vi "Process.vi"(0 "reference in":refnum<class "ACIR_EIS.lvclass">, 5 "error in":errorcluster) -> (14 "reference out":refnum<class "ACIR_EIS.lvclass">, 19 "error out":errorcluster)   [LabVIEW 2023, in "ACIR_EIS.lvclass"]
uses:
  ACIR_EIS.lvclass
  ACIR_EIS.lvclass/ACIR_EIS.ctl
  <vilib>/Utility/SystemLogging/NI_SystemLogging.lvlib
  EIS Mode.ctl
  EIS Parameters.ctl
  Logger_class/Logger.lvclass
  <userlib>/_OpenG.lib/time/time.llb/openg_time.lvlib
  <vilib>/Utility/NIReport.llb/NI_report.lvclass
  <vilib>/Utility/NIReport.llb/Report Type.ctl
  <vilib>/Utility/NIReport.llb/NI_ReportGenerationCore.lvlib
  builds/PowerModuleInterface/PowerModuleInterface.lvlibp/Classes/PowerModule_interface/PowerModuleInterface.lvclass
  <vilib>/printing/OpenHTMLReport.llb/Open HTML Report in Browser (Refnum).vi
panel:
  out "Last Command":string
  out "error info":errorcluster
  in  "Save EIS Report":bool
  in  "EIS Tab Control":T1(tab)
  out "EIS Parameters":T3={"EIS Mode"=2, "EIS DC Potential"=650.0, "EIS Start Frequency"=1000.0, "EIS Stop Frequency"=500.0, "EIS Delta Frequency"=100.0, "EIS DC Current"=0.0, "AC Signal (mV/mA RMS)"=20.0, "Cycles at Frequency"=5.0, "EIS AC Step Delay"=1.0} {"EIS Mode" items=["Voltage (PEIS)"=1, "Current (GEIS)"=2]}
  out "EIS Profile":waveform(dbl)[](graph)
  out "Running Status Log":i32(listbox) caption="TEST SERVER LOG"
  out "EIS Step":dbl[][](graph)
  out "EIS Nyquist":cluster{dbl[], dbl[]}(graph)
  out "EIS Phase":cluster{dbl[], dbl[]}(graph)
  out "EIS Magnitude":cluster{dbl[], dbl[]}(graph)
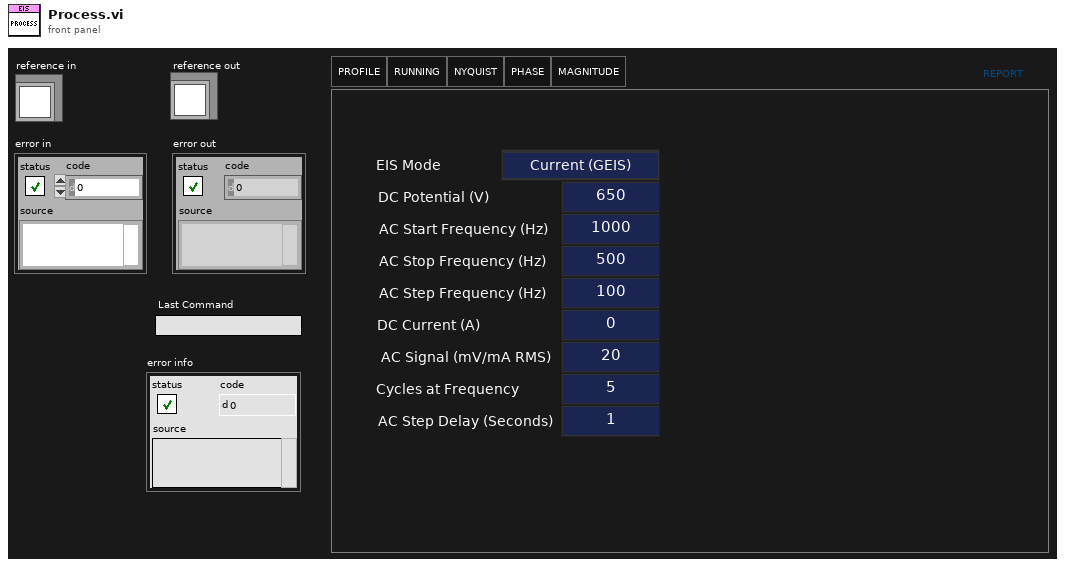
[diagram p1: front panel]
types:
  T1 = enum32{"PARAM", "PROFILE", "RUNNING", "NYQUIST", "PHASE", "MAGNITUDE"}
  T2 = typedef "ACIR_EIS.lvclass/EIS Mode.ctl" = u16
  T3 = cluster{"EIS Mode":T2, "EIS DC Potential":dbl, "EIS Start Frequency":dbl, "EIS Stop Frequency":dbl, "EIS Delta Frequency":dbl, "EIS DC Current":dbl, "AC Signal (mV/mA RMS)":dbl, "Cycles at Frequency":dbl, "EIS AC Step Delay":dbl}
  T4 = typedef "ACIR_EIS.lvclass/EIS Parameters.ctl" = cluster{"EIS Mode":T2, "EIS DC Potential":dbl, "EIS Start Frequency":dbl, "EIS Stop Frequency":dbl, "EIS Delta Frequency":dbl, "EIS DC Current":dbl, "AC Signal (mV/mA RMS)":dbl, "Cycles at Frequency":dbl, "EIS AC Step Delay":dbl}
  T5 = cluster{"Core":cluster{"Timeout":i32, "Events":cluster{"EventsToProcess":refnum<event-registration>}, "EventFromProcess":refnum<user-event>, "ProcessSyncQueue":refnum<queue>, "QueueFromProcess":refnum<queue>, "Command":string, "Data":variant}, "EIS Parameters":T4, "Profile Complete Event":refnum<user-event>, "EIS Profile State":enum16{"Idle", "Start", "Run", "Stop"}, "EIS TDMS Path":path, "Logger":refnum<class "Logger.lvclass">, "Power Module":refnum<class "PowerModuleInterface.lvclass">, "Voltage Profile":waveform(dbl)[], "Current Profile":waveform(dbl)[], "Next Step Timestamp":dbl, "Profile Index":i64, "Frequencies":dbl[]}
  T6 = enum8{"Enabled", "Disabled", "Disabled and Grayed Out"}
  T7 = typedef "NI_ReportGenerationCore.lvlib/Report Type.ctl" = enum16{"HTML", "Word", "Excel"}
  T8 = enum32{"Invalid", "Standard", "Closed", "Hidden", "Minimized", "Maximized"}
  T9 = cluster{"EventsToProcess":refnum<event-registration>}
  T10 = typedef "PowerModuleInterface.lvlibp/PowerModuleInterface.lvclass/Measurements.ctl" = cluster{"measured voltage (V)":dbl, "measured current (A)":dbl, "setpoint voltage (V)":dbl, "setpoint current (A)":dbl, "timestamp":dbl}
  T11 = typedef "ACIR_EIS.lvclass/ObjectAttributes.ctl" = cluster{"EIS Parameters":T4, "Logger":refnum<class "Logger.lvclass">, "Power Module":refnum<class "PowerModuleInterface.lvclass">}
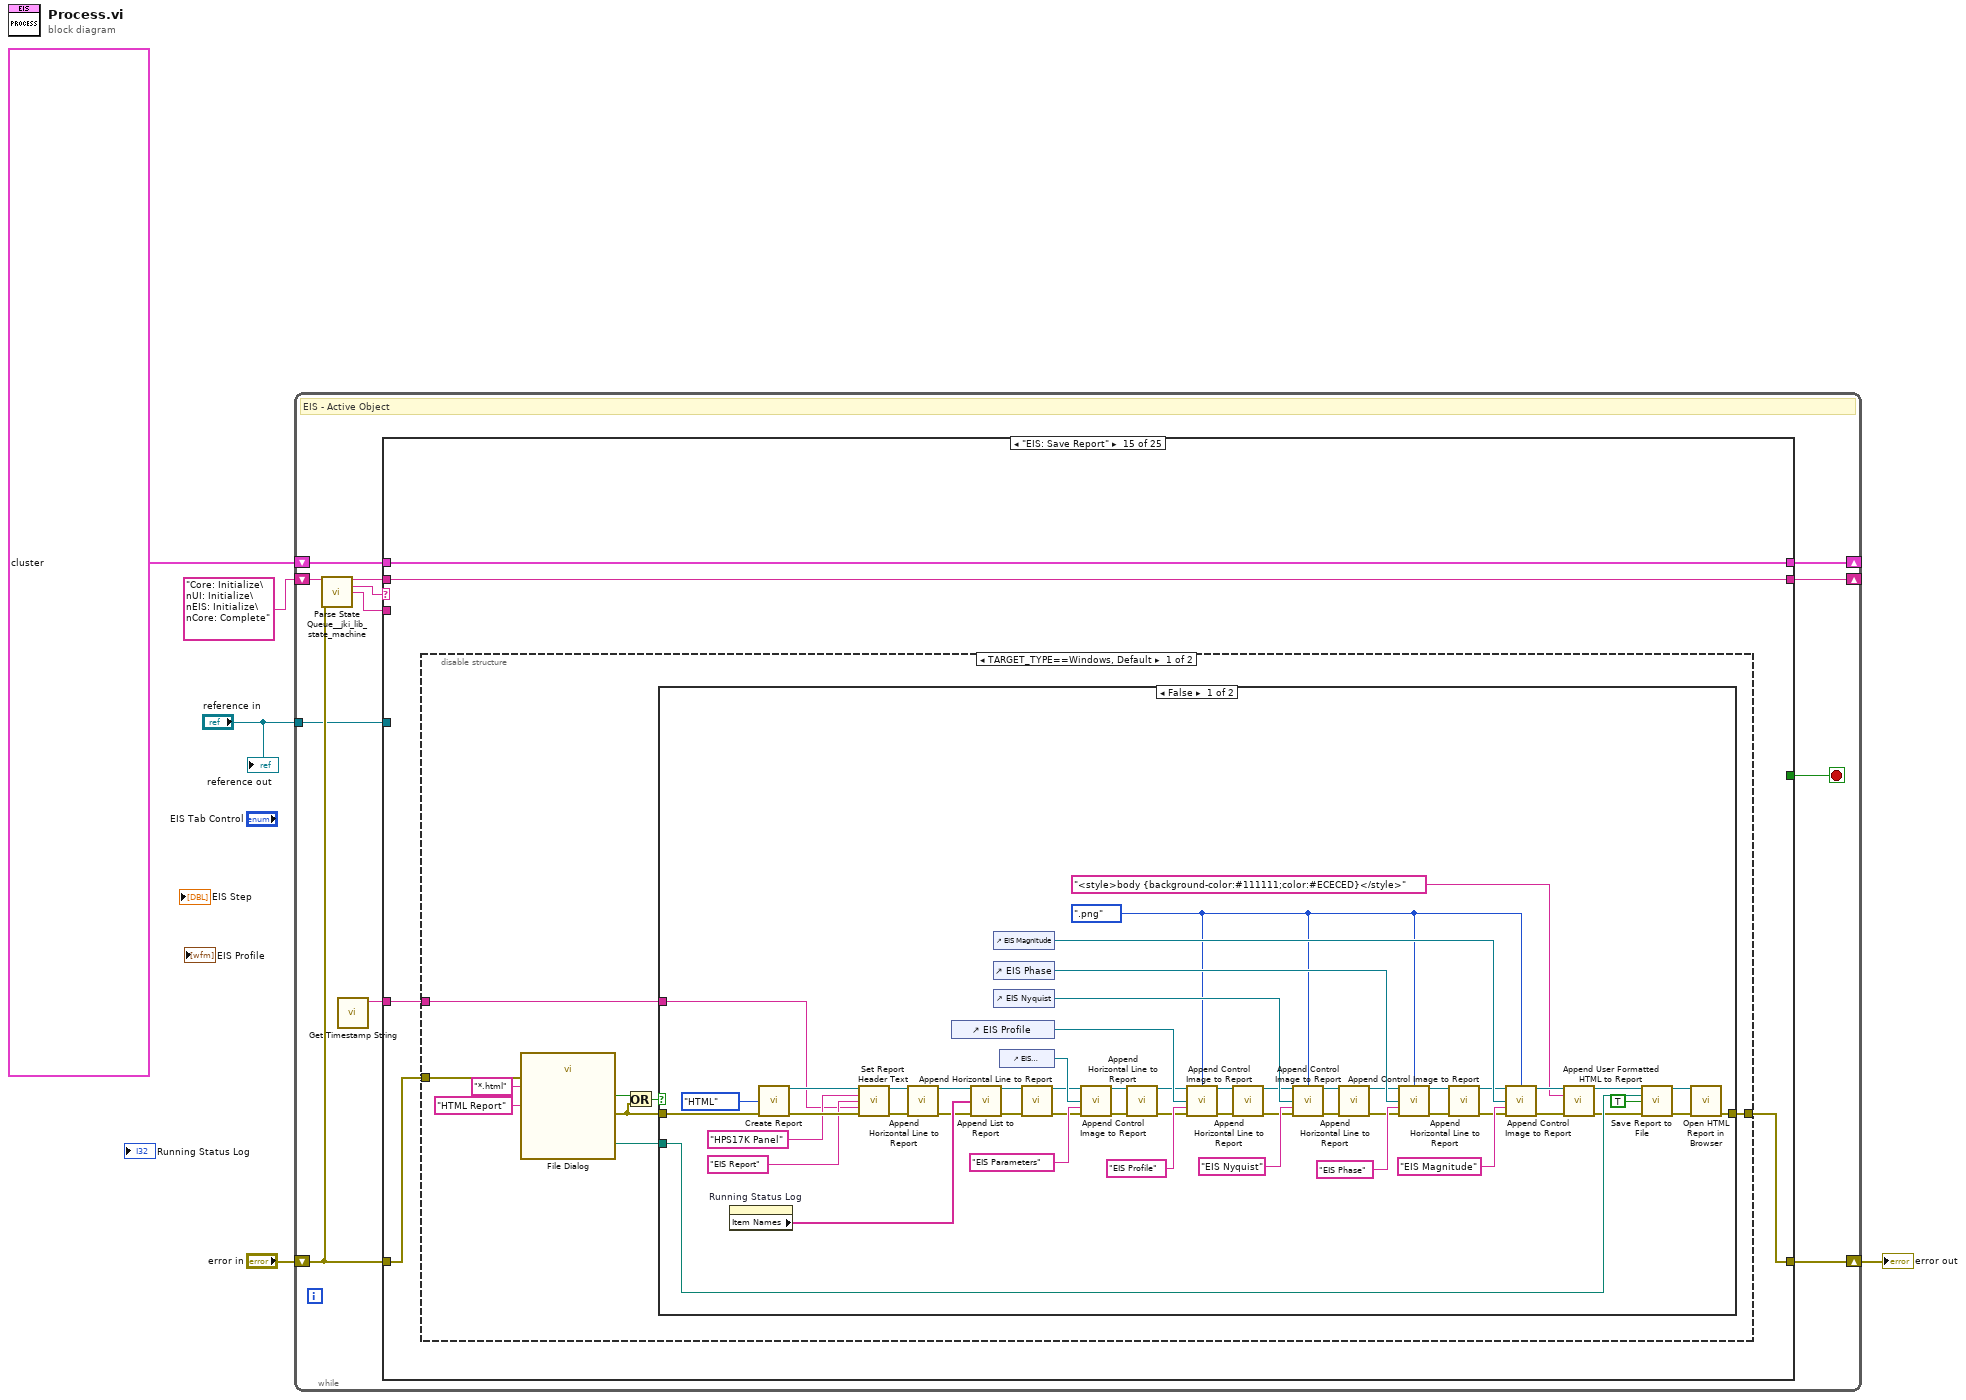
[diagram p0: block diagram]
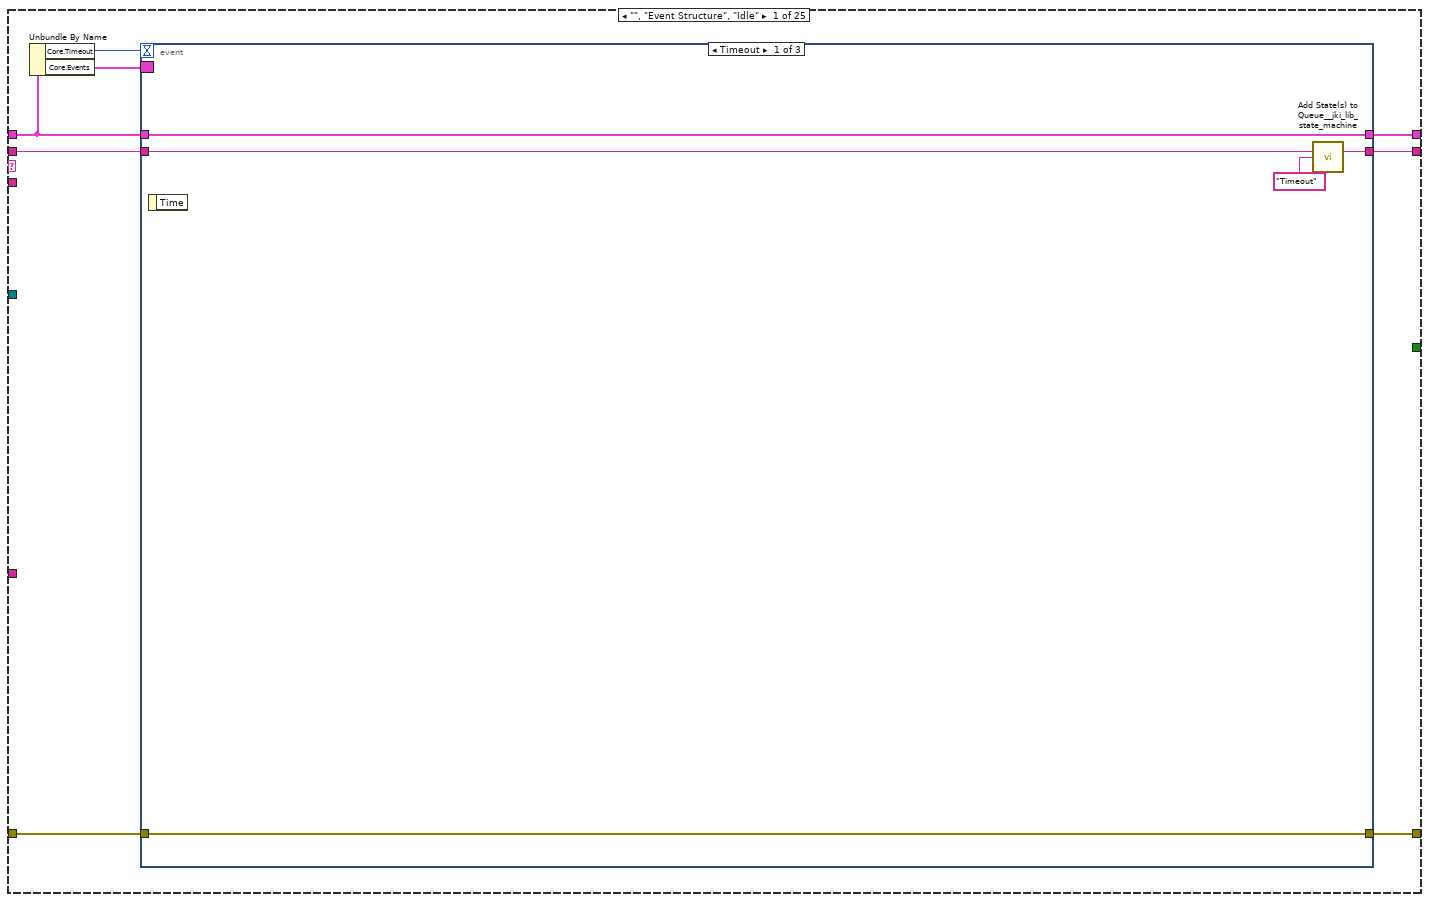
[diagram p2: hidden frame]
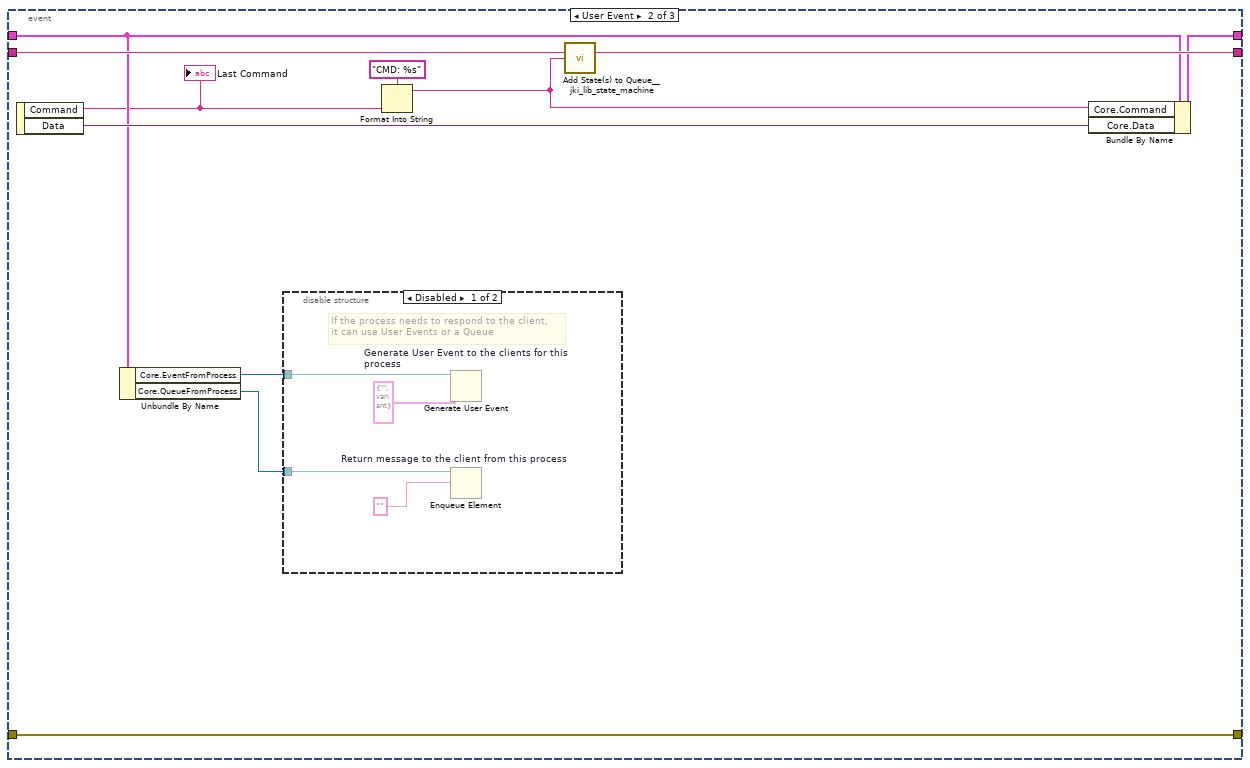
[diagram p3: hidden frame]
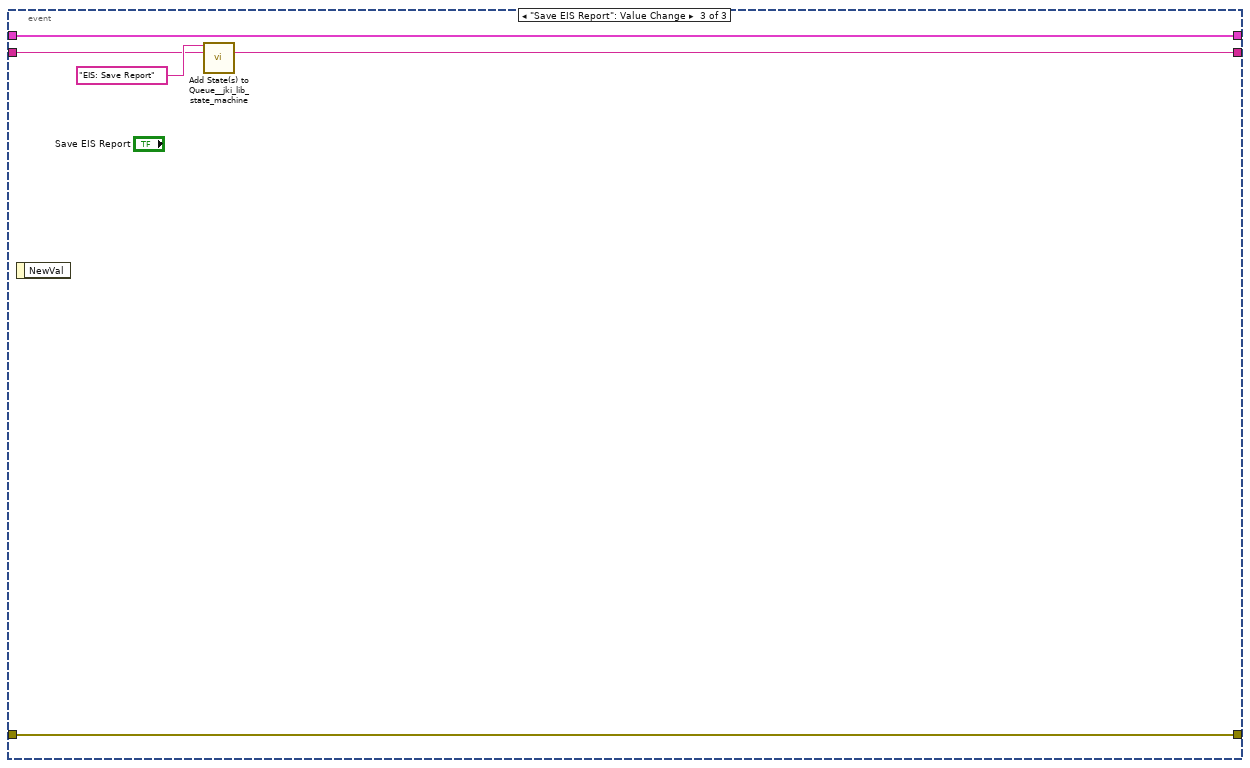
[diagram p5: hidden frame]
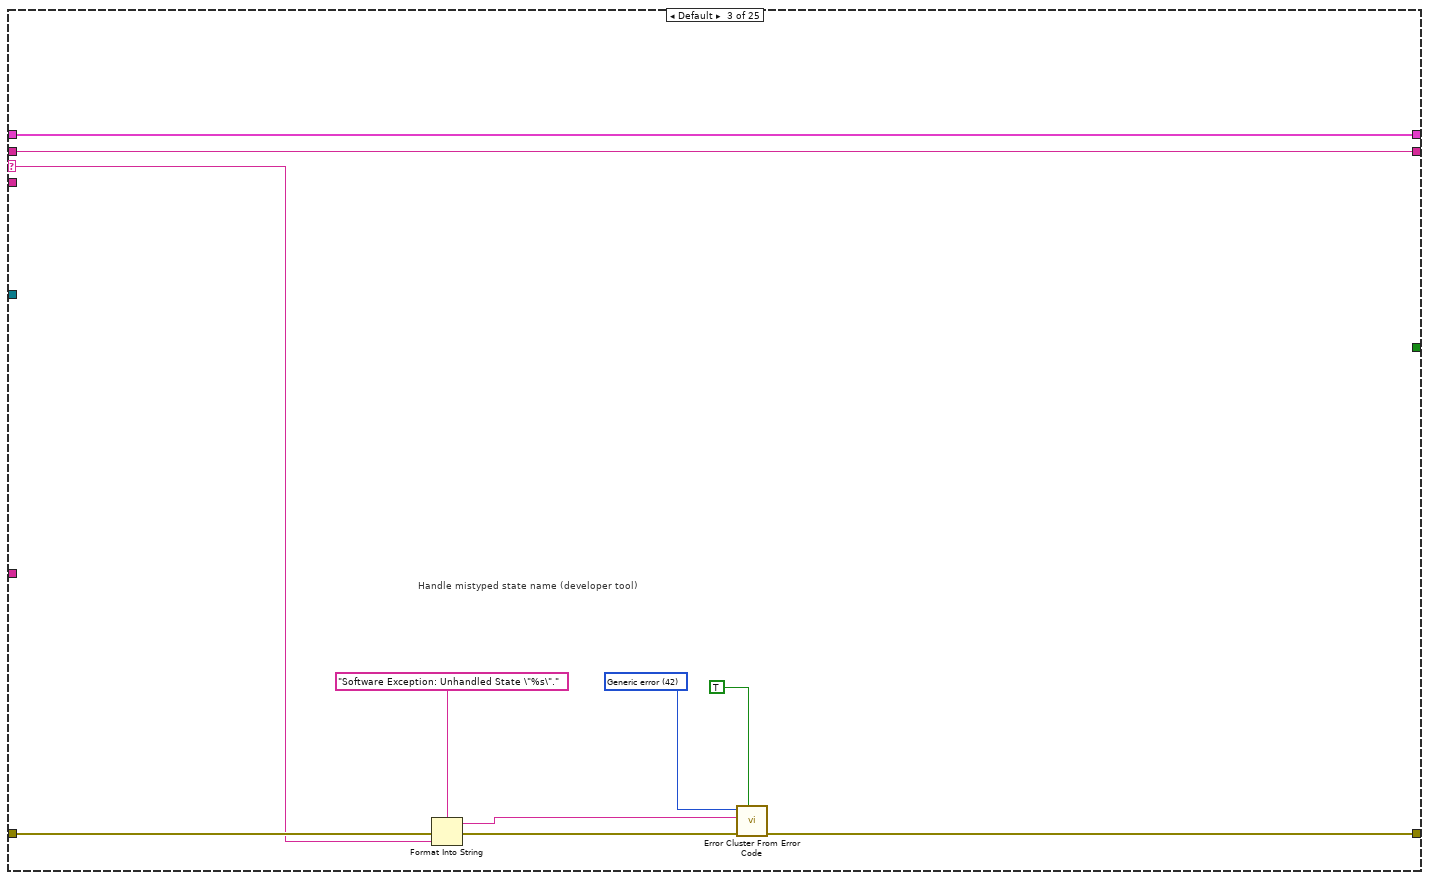
[diagram p7: hidden frame]
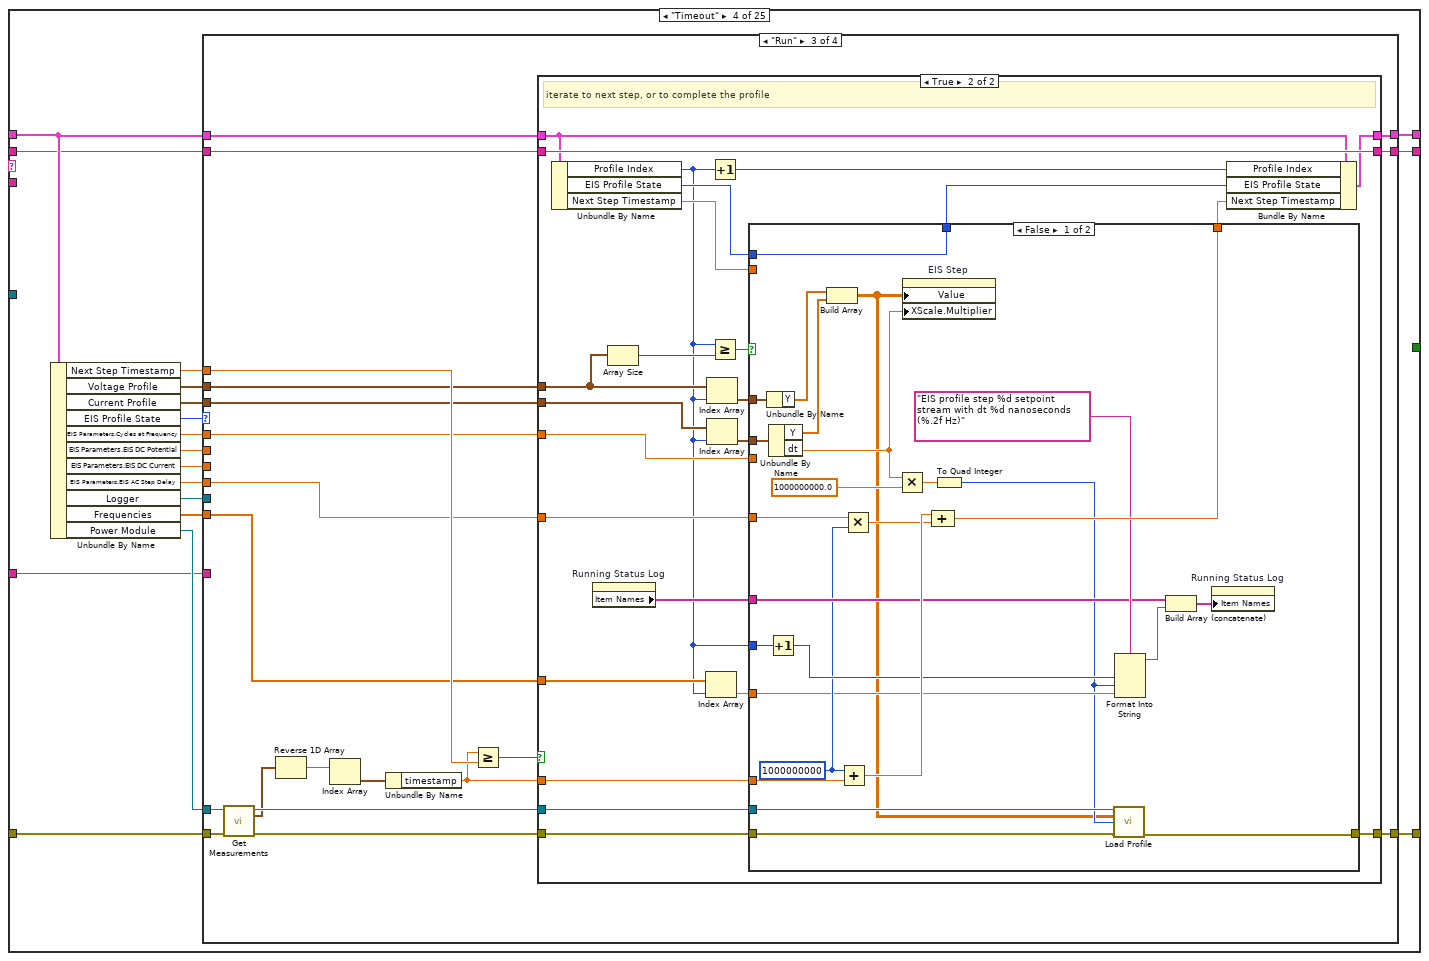
[diagram p8: hidden frame]
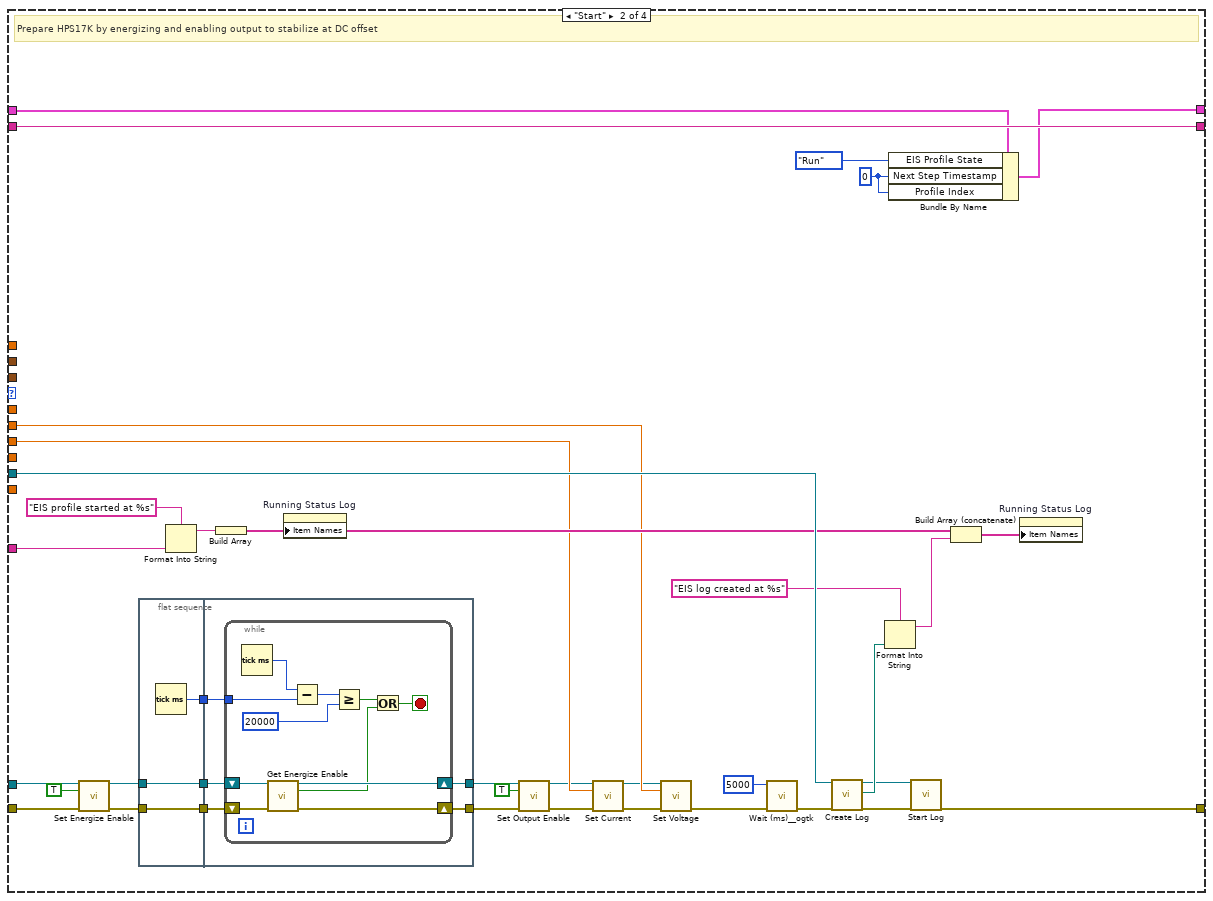
[diagram p10: hidden frame]
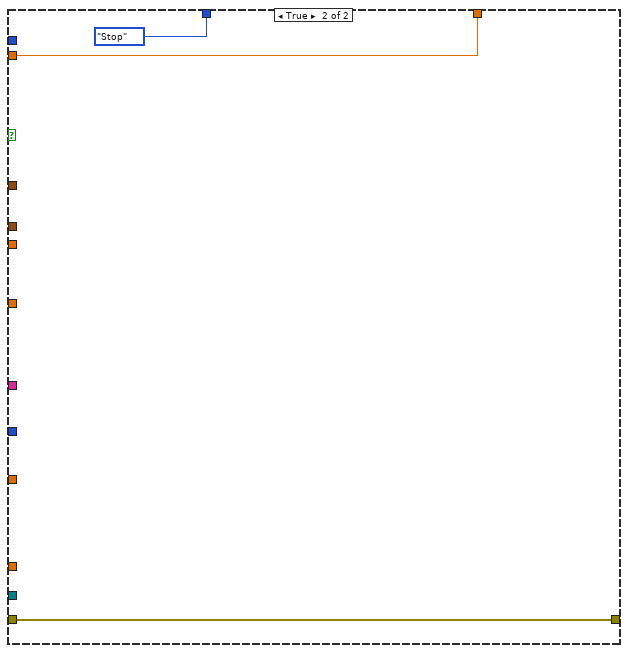
[diagram p12: hidden frame]
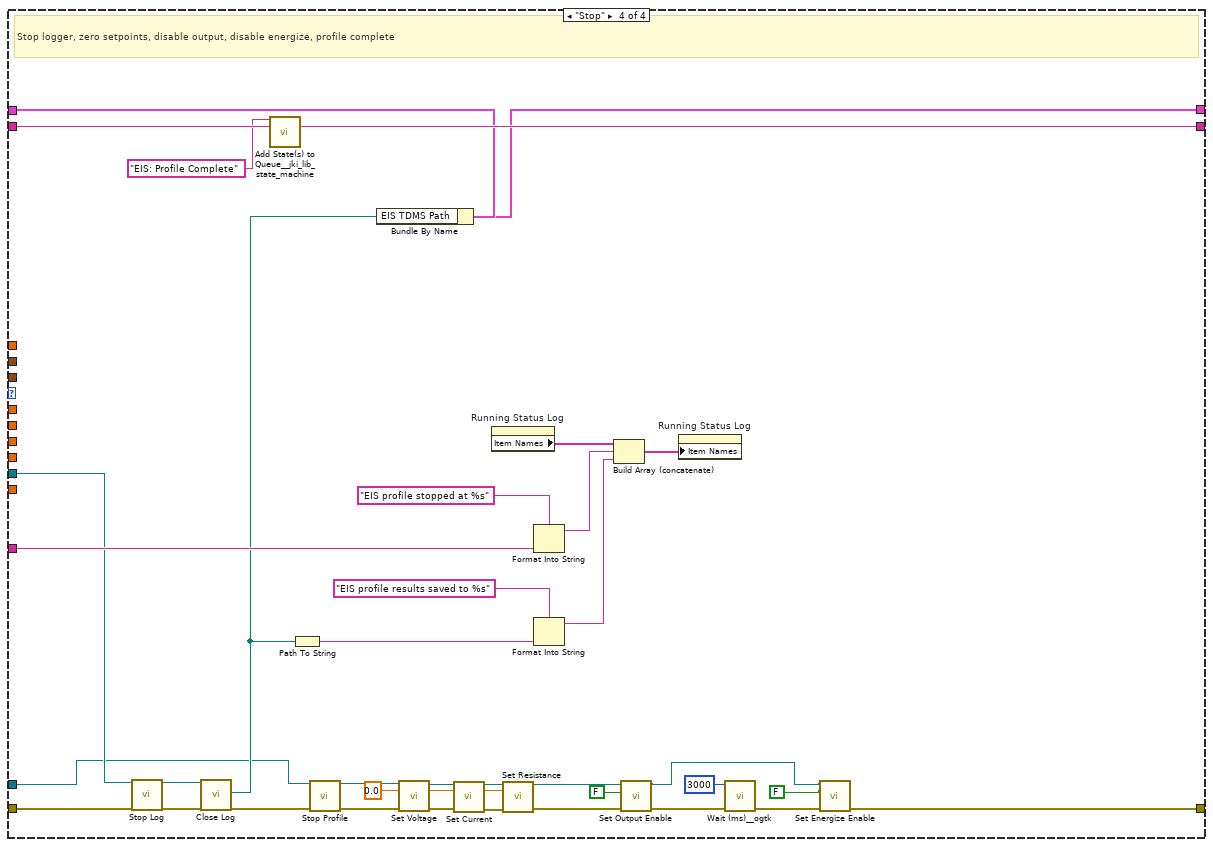
[diagram p13: hidden frame]
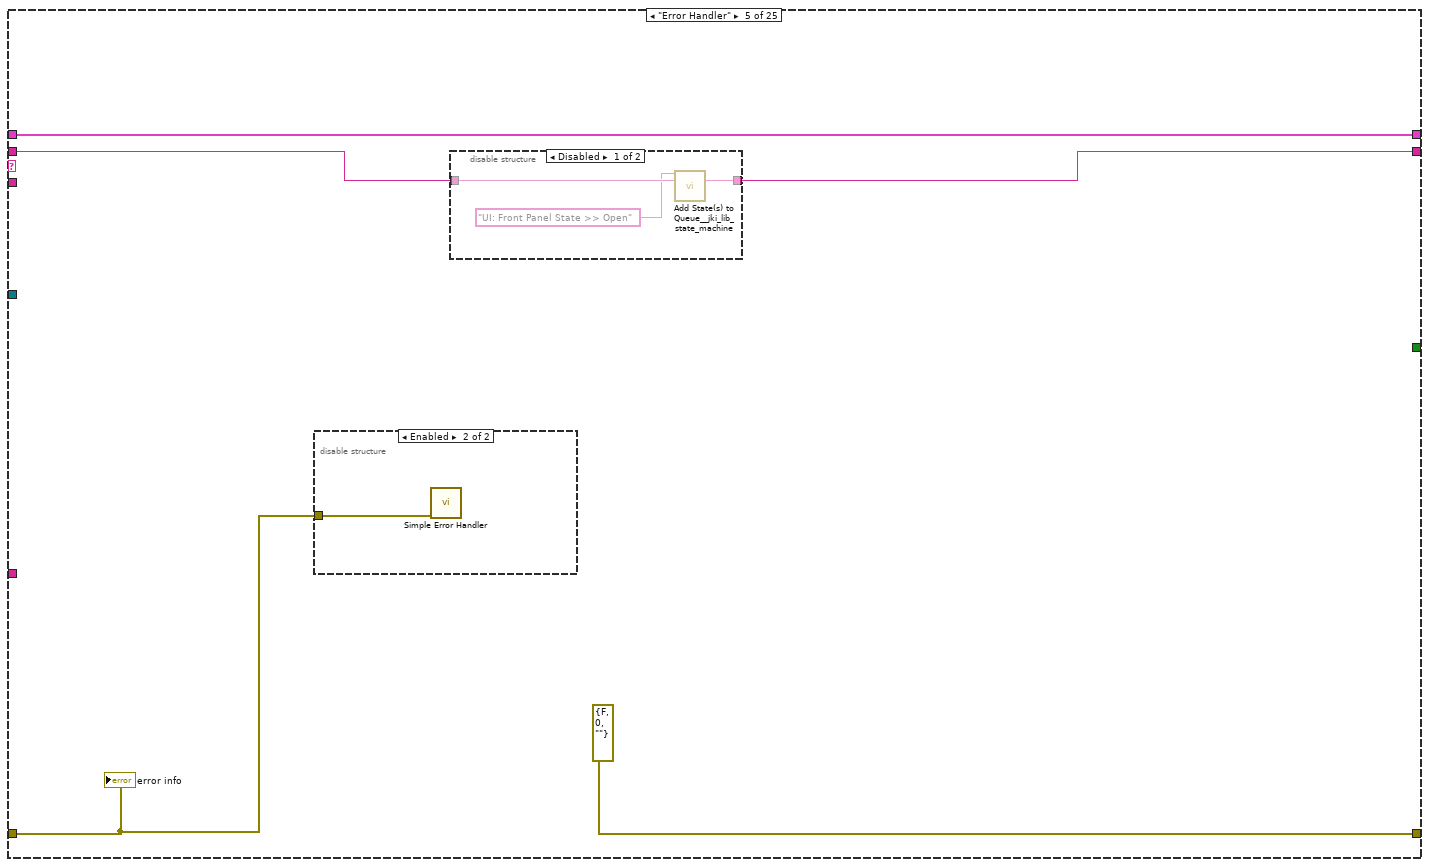
[diagram p14: hidden frame]
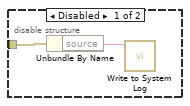
[diagram p16: hidden frame]
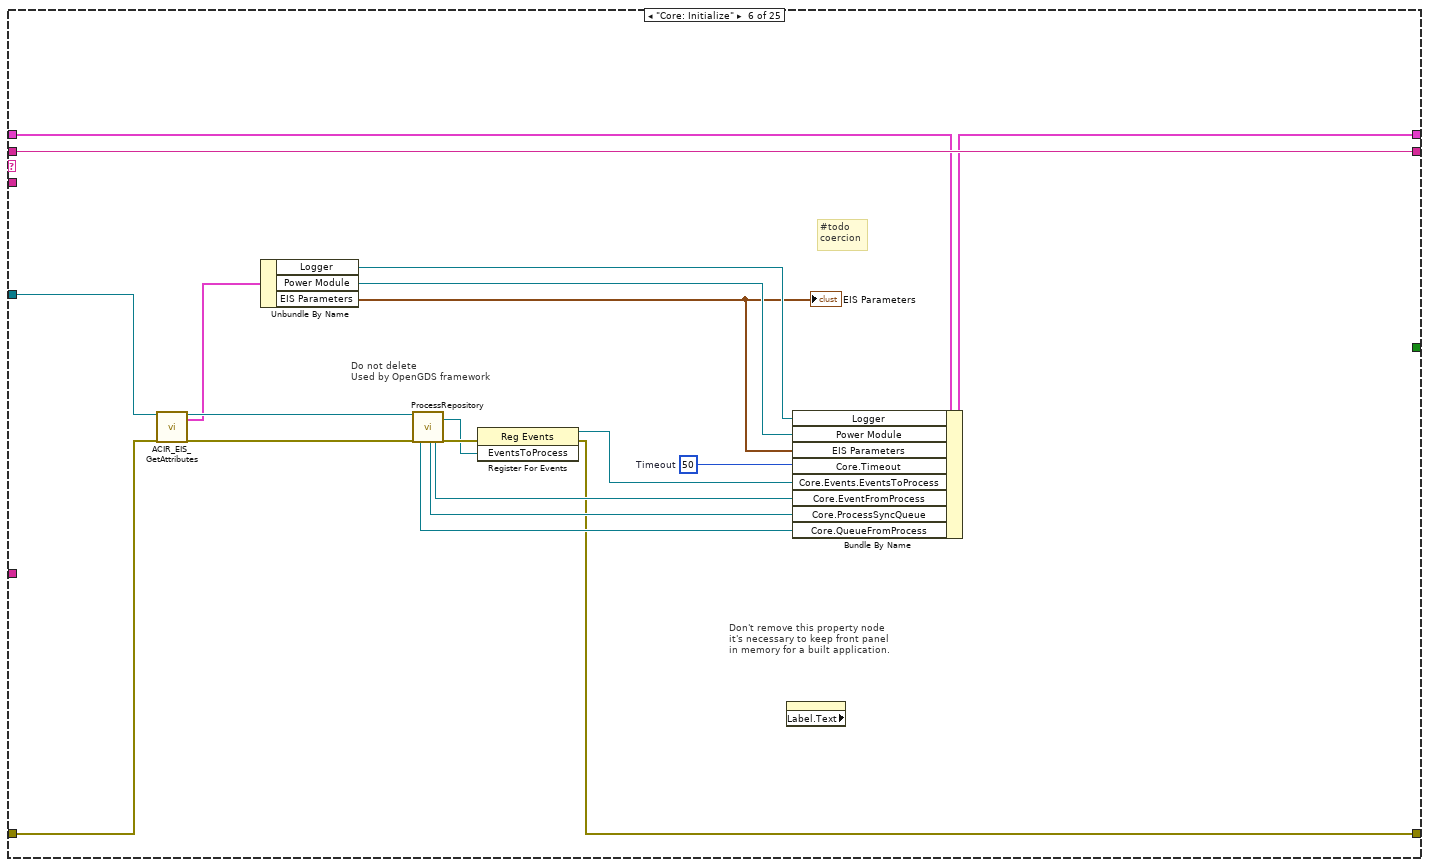
[diagram p17: hidden frame]
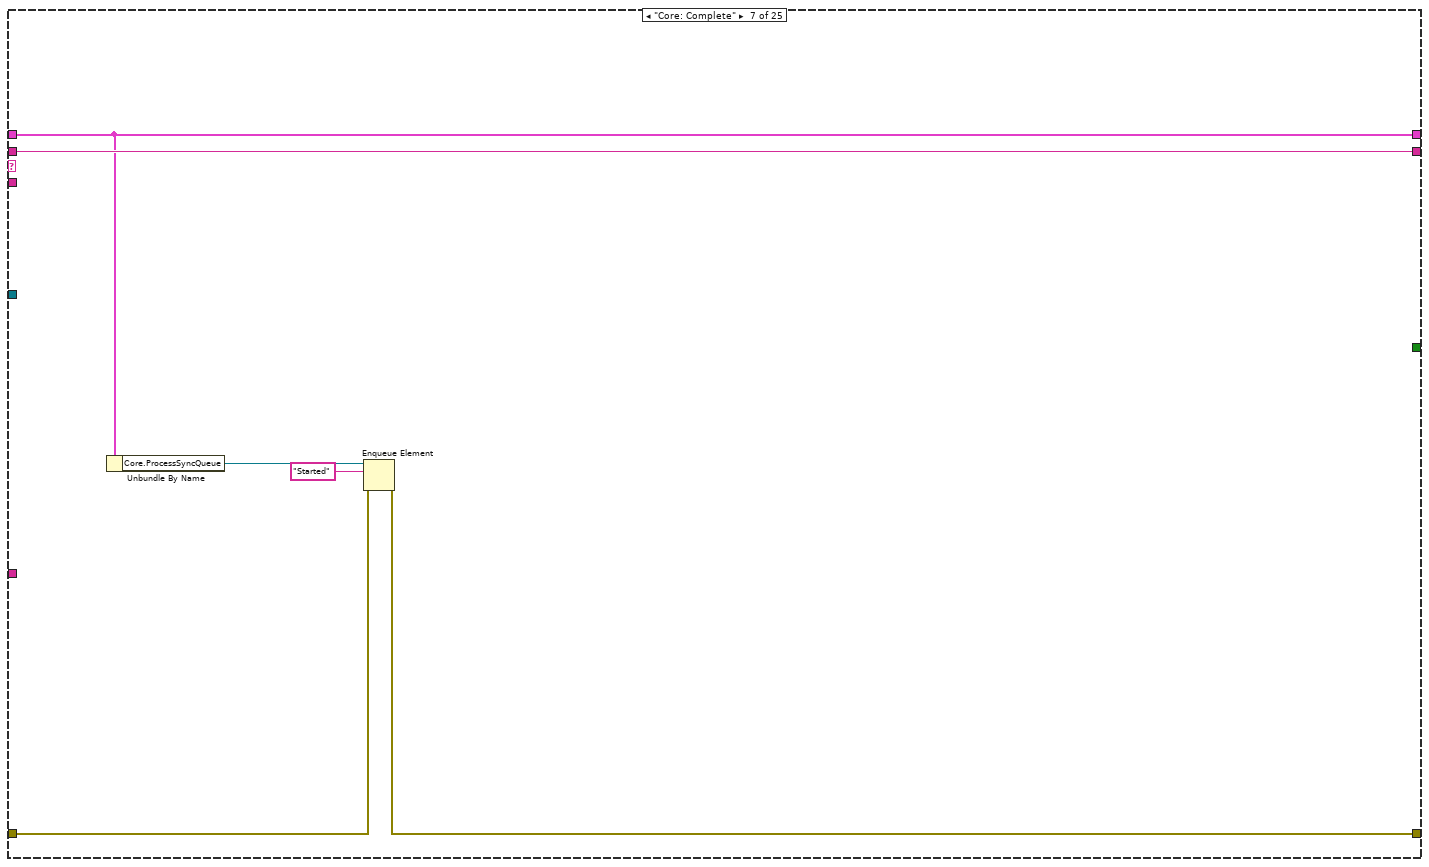
[diagram p18: hidden frame]
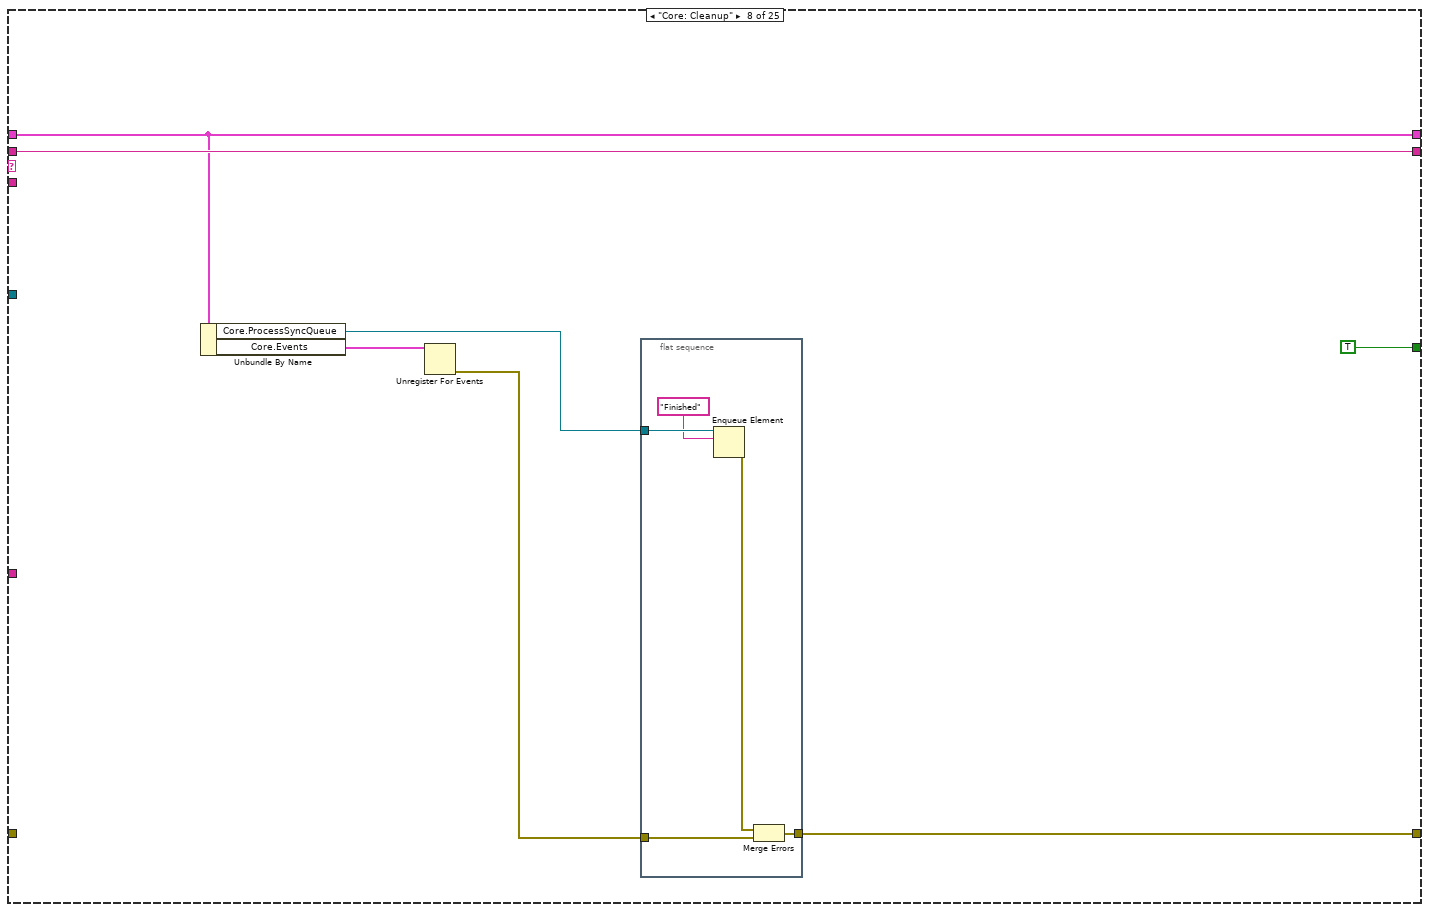
[diagram p19: hidden frame]
diagram:
  n1 = while {
    shift-right: [w16] -> w4
    shift-left: "error in" -> [w17]
    shift-right: [w9] -> _
    shift-left: "Core: Initialize\nUI: Initialize\nEIS: Initialize\nCore: Complete" ("States Out") -> [w12]
    shift-right: [w15] -> _
    shift-left: T5 {"Core"={"Timeout"=-1, "Events"={"EventsToProcess"=refnum}, "EventFromProcess"=refnum, "ProcessSyncQueue"=refnum, "QueueFromProcess"=refnum, "Command"="", "Data"=variant}, "EIS Parameters"={"EIS Mode"=2, "EIS DC Potential"=650.0, "EIS Start Frequency"=1000.0, "EIS Stop Frequency"=500.0, "EIS Delta Frequency"=100.0, "EIS DC Current"=0.0, "AC Signal (mV/mA RMS)"=20.0, "Cycles at Frequency"=1000.0, "EIS AC Step Delay"=1.0}, "Profile Complete Event"=refnum, "EIS Profile State"=enum."Idle", "EIS TDMS Path"=path "", "Logger"=refnum, "Power Module"=refnum, "Voltage Profile"=[], "Current Profile"=[], "Next Step Timestamp"=0.0, "Profile Index"=0, "Frequencies"=[]} ("LocalVariables") -> [w14]
    tunnel: "reference in" -> [w7]
    stop <- w8 stop-if-true
    # "EIS - Active Object"
    n2 = call <vilib>:"Parse State Queue__jki_lib_state_machine.vi"("State Queue"=w12, "Error In (no error)"=w17) -> ("Remaining States"=w11:string, "Current State"=w13:string, "Arguments"=w10:string)  [unwired: 11 in]
    n3 = call "Get Timestamp String.vi"() -> ("date/time string"=w6:string)  [unwired: 11 in]
    n4 = case shown="\"EIS: Save Report\"" w13 {
      selector: w13 -> [_ _ w54 _ _ _ _ _ _ _ _ _ _ _ _ _ _ _ _ _ _ _ _ _ _]
      tunnel: w17 -> [w19 w53 w56 w81 w254 w269 w285 _ w304 w315 w322 w327 w334 w346 w352 w421 w422 w450 _ w457 w460 w467 w475 w482 w487]
      tunnel: [w20 w53 w55 w80 errorcluster {"status"=FALSE, "code"=0, "source"=""} ("error constant") w274 w289 w292 w304 w314 w322 w327 w333 w344 w350 w421 w422 w450 w451 w457 w460 w467 w474 w482 w487] -> w16
      tunnel: [w25 w52 w63 w75 w257 w282 w286 w293 w303 w313 w319 w324 w331 w348 w354 w420 w424 w449 w452 w456 w459 w466 w472 w481 w486] -> w15
      tunnel: w14 -> [w21 w52 w63 w76 w257 w281 w286 w293 w303 w309 w320 w325 w332 w348 w354 w420 w424 w449 w452 w456 w459 w466 w473 w481 w486]
      tunnel: w11 -> [w23 w51 w62 w74 w256 w283 w288 w296 w302 w316 w321 w326 w338 w349 w353 w419 w425 w433 w454 w455 _ w465 w470 w480 w484]
      tunnel: w10 -> [_ _ _ _ _ _ _ _ _ _ _ _ _ _ _ _ w423 _ _ _ _ w462 _ _ _]
      tunnel: [w22 w51 w62 w73 w255 w283 w288 w296 w302 w316 w321 w326 w338 w349 w353 w419 w425 w433 w454 w455 "UI: Cleanup\nCore: Cleanup" ("State(s) at Back (\"\")") w464 w469 w479 w483] -> w9
      tunnel: [_ _ _ _ _ _ _ TRUE _ _ _ _ _ _ _ _ _ _ _ _ _ _ _ _ _] -> w8
      tunnel: w7 -> [_ _ _ _ _ w272 _ _ _ _ _ _ _ _ _ _ _ _ _ _ _ _ _ _ _]
      tunnel: w6 -> [_ _ _ w77 _ _ _ _ _ _ _ _ _ _ w351 _ _ _ _ _ _ _ _ _ _]
      frame "", "Event Structure", "Idle" {
        n5 = Unbundle By Name(w21) -> ("Core.Timeout"=w18:i32, "Core.Events"=w24:T9)
        n6 = event shown="[0] Timeout" {
          selector: w24 -> [_ _ _]
          dyn-events: _ -> [_ _ _]
          timeout: w18 -> [_ _ _]
          tunnel: w21 -> [w30 w34 w50]
          tunnel: [w30 w39 w50] -> w25
          tunnel: [w28 w41 w46] -> w22
          tunnel: w23 -> [w29 w40 w47]
          tunnel: [w26 w35 w49] -> w20
          tunnel: w19 -> [w26 w35 w49]
          event Timeout {
            n7 = event-data() -> ()  [unwired: 1 in, 1 out]
            n8 = call <vilib>:"Add State(s) to Queue__jki_lib_state_machine.vi"("State(s) in (\"\")"=w29, "State(s) at Back (\"\")"="Timeout" ("State(s) at Back (\"\")")) -> ("States Out"=w28:string)  [unwired: 13 in]
          }
          event User Event {
            n9 = event-data() -> ("Command"=w32:string, "Data"=w38:variant)  [unwired: 1 in]
            "Last Command" <- w32
            n10 = Unbundle By Name(w34) -> ("Core.EventFromProcess"=w37:refnum<user-event>, "Core.QueueFromProcess"=w36:refnum<queue>)
            n11 = disable-structure shown="Disabled" {
              disable-tunnel: w37 -> [w45 _]
              disable-tunnel: w36 -> [w44 _]
              frame Disabled {
                # "If the process needs to respond to the client,\nit can use User Events or a Queue"
                n12 = Generate User Event "Generate User Event to the clients for this process"(user event=w45, event data cluster=cluster{"Command":string, "Data":variant} {"Command"="", "Data"=variant} ("event data")) -> ()  [unwired: 2 in, 2 out]
                n13 = Enqueue Element "Return message to the client from this process"(queue=w44, element="") -> ()  [unwired: 2 in, 3 out]
              }
              frame Enabled {
              }
            }
            n14 = Format Into String(format string="CMD: %s", w32) -> (resulting string=w31:string)  [unwired: 2 in, 1 out]
            n15 = call <vilib>:"Add State(s) to Queue__jki_lib_state_machine.vi"("State(s) in (\"\")"=w40, "State(s) at Back (\"\")"=w31) -> ("States Out"=w41:string)  [unwired: 13 in]
            n16 = Bundle By Name(cluster=w34, "Core.Command"=w31, "Core.Data"=w38) -> (w39:T5)
          }
          event "Save EIS Report": Value Change {
            n17 = event-data() -> ()  [unwired: 1 in, 1 out]
            n18 = call <vilib>:"Add State(s) to Queue__jki_lib_state_machine.vi"("State(s) in Front (\"\")"="EIS: Save Report" ("State(s) in Front (\"\")"), "State(s) in (\"\")"=w47) -> ("States Out"=w46:string)  [unwired: 13 in]
          }
        }
      }
      frame "---------- Core ----------" {
      }
      frame Default {
        w60 = 42 items=["No error", "Argument error", "Memory is full", "Out of zone", "End of file", "File already open", "Generic file I/O error", "File not found", "File permission error", "Disk is full", "Duplicate path", "Too many files open", "System feature not enabled", "Resource file not found", "Cannot add resource", "Resource not found", "Image not found", "Image memory error", "Pen does not exist", "Config type invalid", "Config token not found", "Config parse error", "Config memory error", "Bad external code format", "Bad external code offset", "External code not present", "Null window", "Destroy window error", "Null menu", "Print aborted", "Bad print record", "Print driver error", "Windows error during printing", "Memory error during printing", "Print dialog error", "Generic print error", "Invalid device refnum", "Device not found", "Device parameter error", "Device unit error", "Cannot open device", "Device call aborted", "Generic error", "Cancelled by user", "Object ID too low", "Object ID too high", "Object not in heap", "Unknown heap", "Unknown object (invalid DefProc)", "Unknown object (DefProc not in table)", "Message out of range", "Invalid (null) method", "Unknown message", "Manager call not supported", "Bad address", "Network operation in progress", "Network operation timed out", "Connection is busy", "Network attribute not supported", "Network error", "Address in use", "System out of memory", "Connection aborted", "Connection refused", "Not connected", "Already connected", "Connection closed", "Initialization error (interapplication manager)", "Bad occurrence", "Wait on unbound occurrence handler", "Occurrence queue overflow", "Datalog type conflict", "Unused", "Unrecognized type (interapplication manager)", "Memory corrupt", "Failed to make temporary DLL", "Old CIN version", "Drag socket not found", "Failed to load drop-object", "Failed to register OLE object", "Failed to release OLE object", "Format specifier type mismatch", "Unknown format specifier", "Too few format specifiers", "Too many format specifiers", "Scan failed", "Newer CIN version", "Error converting to variant", "Runtime menu error", "Password tampered", "Variant attribute not found", "Incompatible variant data type", "Event data is not available", "Event Store is not present", "Occurrence is not found", "Event Queue is not created", "Event info is not available", "Refnum passed is NULL", "Error retrieving Class GUID", "Error retrieving CoClass GUID", "Error retrieving TypeLib GUID.", "Bad built application magic bytes.", "Specific driver is different from the specific driver associated with the Logical Name.", "There is no session opened to the class driver.", "Max Error", "MAX - Error with config objects", "MAX - Error loading configuration", "MAX - Group not supported"]
        # "Handle mistyped state name (developer tool)"
        n19 = Format Into String(format string="Software Exception: Unhandled State \"%s\"." ("message"), error in=w56, w54) -> (resulting string=w59:string, error out=w58:errorcluster)  [unwired: 1 in]
        n20 = call <vilib>:"Error Cluster From Error Code.vi"("show call chain? (False)"=TRUE, "error in (no error)"=w58, "error message (\"\")"=w59, "error code (0)"=w60) -> ("error out"=w55:errorcluster)  [unwired: 5 in]
      }
      frame "Timeout" {
        n21 = Unbundle By Name(w76) -> ("Next Step Timestamp"=w69:dbl, "Voltage Profile"=w70:waveform(dbl)[], "Current Profile"=w71:waveform(dbl)[], "EIS Profile State"=w79:enum16{"Idle", "Start", "Run", "Stop"}, "EIS Parameters.Cycles at Frequency"=w65:dbl, "EIS Parameters.EIS DC Potential"=w66:dbl, "EIS Parameters.EIS DC Current"=w72:dbl, "EIS Parameters.EIS AC Step Delay"=w67:dbl, "Logger"=w68:refnum<class "Logger.lvclass">, "Frequencies"=w64:dbl[], "Power Module"=w78:refnum<class "PowerModuleInterface.lvclass">)
        n22 = case shown="\"Run\"" w79 {
          tunnel: w81 -> [w84 w97 w147 w244]
          tunnel: [w84 w110 w151 w232] -> w80
          tunnel: w78 -> [_ w96 w146 w226]
          tunnel: w68 -> [_ w121 _ w241]
          tunnel: w77 -> [_ w116 _ w248]
          tunnel: w76 -> [w83 w108 w158 w239]
          tunnel: [w83 w107 w157 w238] -> w75
          tunnel: w74 -> [w82 w109 w156 w247]
          tunnel: [w82 w109 w155 w245] -> w73
          tunnel: w72 -> [_ w98 _ _]
          tunnel: w66 -> [_ w101 _ _]
          tunnel: w71 -> [_ _ w152 _]
          tunnel: w70 -> [_ _ w153 _]
          tunnel: w69 -> [_ _ w160 _]
          tunnel: w67 -> [_ _ w150 _]
          tunnel: w65 -> [_ _ w149 _]
          tunnel: w64 -> [_ _ w148 _]
          frame "Idle", Default {
            # "do nothing"
          }
          frame "Start" {
            w105 = i64 0 ("Next Step Timestamp")
            # "Prepare HPS17K by energizing and enabling output to stabilize at DC offset"
            n23 = call-dynamic "Set Energize Enable.vi"("object in"=w96, "energize"=TRUE, "Error In"=w97) -> ("object out"=w93:refnum<class "PowerModuleInterface.lvclass">, "Error Out"=w94:errorcluster)  [unwired: 11 in]
            n24 = flat-sequence {
              tunnel: w93 -> [w123]
              tunnel: w94 -> [w124]
              tunnel: [w124] -> w87
              tunnel: [w123] -> w86
              tunnel: [w122] -> w85
              tunnel: [w127] -> w90
              tunnel: [w126] -> w89
              tunnel: w87 -> [w129]
              tunnel: w86 -> [w128]
              tunnel: w85 -> [w125]
              frame #0 {
                n25 = Tick Count (ms)() -> (millisecond timer value=w122:u32)
              }
              frame #1 {
                n26 = while {
                  shift-right: [w137] -> w126
                  shift-left: w129 -> [w140]
                  shift-right: [w138] -> w127
                  shift-left: w128 -> [w139]
                  tunnel: w125 -> [w133]
                  stop <- w135 stop-if-true
                  n27 = Tick Count (ms)() -> (millisecond timer value=w134:u32)
                  n28 = call-dynamic "Get Energize Enable.vi"("object in"=w139, "Error In"=w140) -> ("object out"=w138:refnum<class "PowerModuleInterface.lvclass">, "energized"=w136:bool, "Error Out"=w137:errorcluster)  [unwired: 11 in]
                  n29 = Subtract(x=w134, y=w133) -> (x-y=w132:u32)
                  n30 = Greater Or Equal?(x=w132, y=u32 20000 ("timeout (ms)")) -> (x >= y?=w130:bool)
                  n31 = Or(x=w130, y=w136) -> (x .or. y?=w135:bool)
                }
              }
            }
            n32 = Format Into String(format string="EIS profile started at %s", w116) -> (resulting string=w104:string)  [unwired: 2 in, 1 out]
            n33 = Build Array(w104) -> (w103:string[])
            n34 = property on="Running Status Log" class="LstBox (strict)"("Item Names"=w103) -> ()  [unwired: 2 in, 2 out]
            n35 = call-dynamic "Set Output Enable.vi"("object in"=w90, "output"=TRUE, "Error In"=w89) -> ("object out"=w91:refnum<class "PowerModuleInterface.lvclass">, "Error Out"=w92:errorcluster)  [unwired: 11 in]
            n36 = call-dynamic "Set Current.vi"("object in"=w91, "current (A)"=w98, "Error In"=w92) -> ("object out"=w99:refnum<class "PowerModuleInterface.lvclass">, "Error Out"=w100:errorcluster)  [unwired: 11 in]
            n37 = call-dynamic "Set Voltage.vi"("object in"=w99, "voltage (V)"=w101, "Error In"=w100) -> ("Error Out"=w102:errorcluster)  [unwired: 11 in, 1 out]
            n38 = call <userlib>:"Wait (ms)__ogtk.vi"("error in (no error)"=w102, "milliseconds to wait"=u32 5000) -> ("error out"=w120:errorcluster)  [unwired: 8 in, 1 out]
            n39 = call "Create Log.vi"("reference in"=w121, "Error In"=w120) -> ("reference out"=w113:refnum<class "Logger.lvclass">, "created file"=w114:path, "Error Out"=w118:errorcluster)  [unwired: 15 in]
            n40 = Format Into String(format string="EIS log created at %s", w114) -> (resulting string=w112:string)  [unwired: 2 in, 1 out]
            n41 = Bundle By Name(cluster=w108, "EIS Profile State"=enum16{"Idle", "Start", "Run", "Stop"}."Run", "Next Step Timestamp"=w105, "Profile Index"=w105) -> (w107:T5)
            n42 = call "Start Log.vi"("reference in"=w113, "Error In"=w118) -> ("Error Out"=w110:errorcluster)  [unwired: 16 in, 1 out]
            n43 = Build Array (concatenate)(w103, w112) -> (w111:string[])
            n44 = property on="Running Status Log" class="LstBox (strict)"("Item Names"=w111) -> ()  [unwired: 2 in, 2 out]
          }
          frame "Run" {
            n45 = call-dynamic "Get Measurements.vi"("object in"=w146, "Error In"=w147) -> ("object out"=w144:refnum<class "PowerModuleInterface.lvclass">, "measurements"=w143:T10[], "Error Out"=w145:errorcluster)  [unwired: 11 in]
            n46 = Reverse 1D Array(array=w143) -> (reversed array=w142:T10[])
            n47 = Index Array(array=w142) -> (element=w141:T10)  [unwired: 1 in]
            n48 = Unbundle By Name(w141) -> ("timestamp"=w154:dbl)
            n49 = Greater Or Equal?(x=w154, y=w160) -> (x >= y?=w159:bool)
            n50 = case shown="True" w159 {
              tunnel: w158 -> [w163 w186]
              tunnel: [w163 w184] -> w157
              tunnel: w156 -> [w162 w187]
              tunnel: [w162 w187] -> w155
              tunnel: w145 -> [w161 w179]
              tunnel: w154 -> [_ w172]
              tunnel: w153 -> [_ w177]
              tunnel: w152 -> [_ w176]
              tunnel: [w161 w178] -> w151
              tunnel: w144 -> [_ w173]
              tunnel: w150 -> [_ w171]
              tunnel: w149 -> [_ w167]
              tunnel: w148 -> [_ w166]
              frame False {
                # "wait until current step is completed, do nothing"
              }
              frame True {
                # "iterate to next step, or to complete the profile"
                n51 = Unbundle By Name(w186) -> ("Profile Index"=w165:i64, "EIS Profile State"=w180:enum16{"Idle", "Start", "Run", "Stop"}, "Next Step Timestamp"=w169:dbl)
                n52 = property on="Running Status Log" class="LstBox (strict)"() -> ("Item Names"=w168:string[])  [unwired: 2 in, 2 out]
                n53 = Array Size(array=w177) -> (size(s)=w185:i32)
                n54 = Index Array(array=w166, index=w165) -> (element=w164:dbl)
                n55 = Index Array(array=w177, index=w165) -> (element=w175:waveform(dbl))
                n56 = Index Array(array=w176, index=w165) -> (element=w174:waveform(dbl))
                n57 = Increment(x=w165) -> (x+1=w183:i64)
                n58 = Greater Or Equal?(x=w165, y=w185) -> (x >= y?=w182:bool)
                n59 = case shown="False" w182 {
                  tunnel: [w213 enum16{"Idle", "Start", "Run", "Stop"}."Stop" ("EIS Profile State")] -> w181
                  tunnel: w180 -> [w213 _]
                  tunnel: w179 -> [w193 w215]
                  tunnel: [w192 w215] -> w178
                  tunnel: w175 -> [w212 _]
                  tunnel: w174 -> [w211 _]
                  tunnel: w173 -> [w194 _]
                  tunnel: w172 -> [w210 _]
                  tunnel: w171 -> [w209 _]
                  tunnel: [w207 w214] -> w170
                  tunnel: w169 -> [_ w214]
                  tunnel: w168 -> [w203 _]
                  tunnel: w165 -> [w202 _]
                  tunnel: w167 -> [_ _]
                  tunnel: w164 -> [w195 _]
                  frame False {
                    w199 = i64 1000000000 ("x")
                    n60 = Unbundle By Name(w212) -> ("Y"=w190:dbl[])
                    n61 = Increment(x=w202) -> (x+1=w201:i64)
                    n62 = Unbundle By Name(w211) -> ("Y"=w189:dbl[], "dt"=w196:dbl)
                    n63 = Build Array(w190, w189) -> (w188:dbl[][])
                    n64 = Add(x=w199, y=w210) -> (x+y=w208:dbl)
                    n65 = Multiply(x=w209, y=w199) -> (x*y=w200:dbl)
                    n66 = Multiply(x=w196, y=1000000000.0) -> (x*y=w197:dbl)
                    n67 = property on="EIS Step" class="WFGraph (strict)"("Value"=w188, "XScale.Multiplier"=w196) -> ()  [unwired: 2 in, 2 out]
                    n68 = Compound Arithmetic op=ADD(w208, w200) -> (w207:dbl)
                    n69 = To Quad Integer(1:w197) -> (0:w191:i64)
                    n70 = call-dynamic "Load Profile.vi"("object in"=w194, "profile"=w188, "step dt"=w191, "Error In"=w193) -> ("Error Out"=w192:errorcluster)  [unwired: 10 in, 1 out]
                    n71 = Format Into String(format string="EIS profile step %d setpoint stream with dt %d nanoseconds (%.2f Hz)", w201, w191, w195) -> (resulting string=w206:string)  [unwired: 2 in, 1 out]
                    n72 = Build Array (concatenate)(w203, w206) -> (w205:string[])
                    n73 = property on="Running Status Log" class="LstBox (strict)"("Item Names"=w205) -> ()  [unwired: 2 in, 2 out]
                  }
                  frame True {
                  }
                }
                n74 = Bundle By Name(cluster=w186, "Profile Index"=w183, "EIS Profile State"=w181, "Next Step Timestamp"=w170) -> (w184:T5)
              }
            }
          }
          frame "Stop" {
            w217 = 0.0 ("voltage (V)")
            # "Stop logger, zero setpoints, disable output, disable energize, profile complete"
            n75 = call "Stop Log.vi"("reference in"=w241, "Error In"=w244) -> ("reference out"=w242:refnum<class "Logger.lvclass">, "Error Out"=w243:errorcluster)  [unwired: 16 in]
            n76 = call "Close Log.vi"("reference in"=w242, "Error In"=w243) -> ("log file path"=w234:path, "Error Out"=w227:errorcluster)  [unwired: 15 in, 1 out]
            n77 = call <vilib>:"Add State(s) to Queue__jki_lib_state_machine.vi"("State(s) in Front (\"\")"="EIS: Profile Complete" ("State(s) in Front (\"\")"), "State(s) in (\"\")"=w247) -> ("States Out"=w245:string)  [unwired: 13 in]
            n78 = Path To String(path=w234) -> (string=w236:string)
            n79 = call-dynamic "Stop Profile.vi"("object in"=w226, "Error In"=w227) -> ("object out"=w218:refnum<class "PowerModuleInterface.lvclass">, "Error Out"=w225:errorcluster)  [unwired: 12 in]
            n80 = Bundle By Name(cluster=w239, "EIS TDMS Path"=w234) -> (w238:T5)
            n81 = call-dynamic "Set Voltage.vi"("object in"=w218, "voltage (V)"=w217, "Error In"=w225) -> ("object out"=w219:refnum<class "PowerModuleInterface.lvclass">, "Error Out"=w224:errorcluster)  [unwired: 11 in]
            n82 = call-dynamic "Set Current.vi"("object in"=w219, "current (A)"=w217, "Error In"=w224) -> ("object out"=w220:refnum<class "PowerModuleInterface.lvclass">, "Error Out"=w223:errorcluster)  [unwired: 11 in]
            n83 = property on="Running Status Log" class="LstBox (strict)"() -> ("Item Names"=w252:string[])  [unwired: 2 in, 2 out]
            n84 = call-dynamic "Set Resistance.vi"("object in"=w220, "resistance (Ohm)"=w217, "Error In"=w223) -> ("object out"=w221:refnum<class "PowerModuleInterface.lvclass">, "Error Out"=w222:errorcluster)  [unwired: 11 in]
            n85 = Format Into String(format string="EIS profile stopped at %s", w248) -> (resulting string=w251:string)  [unwired: 2 in, 1 out]
            n86 = Format Into String(format string="EIS profile results saved to %s", w236) -> (resulting string=w235:string)  [unwired: 2 in, 1 out]
            n87 = Build Array (concatenate)(w252, w251, w235) -> (w250:string[])
            n88 = call-dynamic "Set Output Enable.vi"("object in"=w221, "output"=FALSE ("enabled output"), "Error In"=w222) -> ("object out"=w229:refnum<class "PowerModuleInterface.lvclass">, "Error Out"=w230:errorcluster)  [unwired: 11 in]
            n89 = property on="Running Status Log" class="LstBox (strict)"("Item Names"=w250) -> ()  [unwired: 2 in, 2 out]
            n90 = call <userlib>:"Wait (ms)__ogtk.vi"("error in (no error)"=w230, "milliseconds to wait"=u32 3000) -> ("error out"=w233:errorcluster)  [unwired: 8 in, 1 out]
            n91 = call-dynamic "Set Energize Enable.vi"("object in"=w229, "energize"=FALSE ("energize (T)"), "Error In"=w233) -> ("Error Out"=w232:errorcluster)  [unwired: 11 in, 1 out]
          }
        }
      }
      frame "Error Handler" {
        n92 = disable-structure shown="Enabled" {
          disable-tunnel: w254 -> [w263 w264]
          frame Disabled {
            n93 = Unbundle By Name(w263) -> ("source"=w262:string)
            n94 = call <vilib>:"Write to System Log.vi"("message"=w262) -> ()  [unwired: 10 in, 1 out]
          }
          frame Enabled {
            n95 = call <vilib>:"Simple Error Handler.vi"("error in (no error)"=w264) -> ()  [unwired: 4 in, 5 out]
          }
        }
        n96 = disable-structure shown="Disabled" {
          disable-tunnel: w256 -> [w260 w261]
          disable-tunnel: [w259 w261] -> w255
          frame Disabled {
            n97 = call <vilib>:"Add State(s) to Queue__jki_lib_state_machine.vi"("State(s) in Front (\"\")"="UI: Front Panel State >> Open" ("State(s) at Back (\"\")"), "State(s) in (\"\")"=w260) -> ("States Out"=w259:string)  [unwired: 13 in]
          }
          frame Enabled {
          }
        }
        "error info" <- w254
      }
      frame "Core: Initialize" {
        w273 = 50  # Timeout
        # "#todo\ncoercion"
        # "Do not delete\nUsed by OpenGDS framework"
        # "Don't remove this property node\nit's necessary to keep front panel\nin memory for a built application."
        # "Template created by VI Technologies"
        n98 = call "ACIR_EIS_GetAttributes.vi"("reference in"=w272, "Error In"=w269) -> ("reference out"=w271:refnum<class "ACIR_EIS.lvclass">, "Data"=w268:T11, "Error Out"=w270:errorcluster)  [unwired: 14 in, 1 out]
        n99 = Unbundle By Name(w268) -> ("Logger"=w266:refnum<class "Logger.lvclass">, "Power Module"=w267:refnum<class "PowerModuleInterface.lvclass">, "EIS Parameters"=w265:T4)
        "EIS Parameters" <- w265
        n100 = call "ProcessRepository.vi"("reference in"=w271, "Error In"=w270) -> ("QueueFromProcess"=w276:refnum<queue>, "ProcessSyncQueue"=w275:refnum<queue>, "EventFromProcess"=w277:refnum<user-event>, "EventsToProcess"=w279:refnum<user-event>, "Error Out"=w280:errorcluster)  [unwired: 10 in, 3 out]
        n101 = register-events(error in=w280, w279) -> (reference out=w278:refnum<event-registration>, error out=w274:errorcluster)  [unwired: 1 in]
        n102 = property on="reference in" class="LVClassControl (strict)" props=["Label", "Text"]() -> ()  [unwired: 2 in, 3 out]
        n103 = Bundle By Name(cluster=w281, "Logger"=w266, "Power Module"=w267, "EIS Parameters"=w265, "Core.Timeout"=w273, "Core.Events.EventsToProcess"=w278, "Core.EventFromProcess"=w277, "Core.ProcessSyncQueue"=w275, "Core.QueueFromProcess"=w276) -> (w282:T5)
      }
      frame "Core: Complete" {
        # "Template created by VI Technologies"
        n104 = Unbundle By Name(w286) -> ("Core.ProcessSyncQueue"=w284:refnum<queue>)
        n105 = Enqueue Element(queue=w284, element="Started", error in (no error)=w285) -> (error out=w289:errorcluster)  [unwired: 1 in, 2 out]
      }
      frame "Core: Cleanup" {
        n106 = Unbundle By Name(w293) -> ("Core.ProcessSyncQueue"=w294:refnum<queue>, "Core.Events"=w291:T9)
        n107 = Unregister For Events(event registration refnum=w291) -> (error out=w290:errorcluster)  [unwired: 1 in]
        n108 = flat-sequence {
          tunnel: [w300] -> w292
          tunnel: w294 -> [w299]
          tunnel: w290 -> [w298]
          frame #0 {
            n109 = Enqueue Element(queue=w299, element="Finished") -> (error out=w301:errorcluster)  [unwired: 2 in, 2 out]
            n110 = Merge Errors(w301, w298) -> (w300:errorcluster)
          }
        }
      }
      frame "---------- EIS ----------" {
      }
      frame "EIS: Initialize" {
        n111 = Unbundle By Name(w309) -> ("EIS Parameters"=w308:T4)
        n112 = call "Generate Profile.vi"("error in (no error)"=w315, "EIS Parameters"=w308) -> ("error out"=w314:errorcluster, "EIS Profile"=w307:waveform(dbl)[], "Voltage Profile out"=w310:waveform(dbl)[], "Current Profile out"=w311:waveform(dbl)[], "Frequencies"=w305:dbl[])  [unwired: 5 in]
        n113 = local write "EIS Tab Control"(T1."PROFILE" ("EIS Tab Control")) -> ()
        n114 = Bundle By Name(cluster=w309, "Frequencies"=w305, "EIS Profile State"=enum16{"Idle", "Start", "Run", "Stop"}."Idle", "Voltage Profile"=w311, "Current Profile"=w310) -> (w313:T5)
        n115 = property on="EIS Profile" class="WFGraph (strict)"("Value"=w307) -> ()  [unwired: 2 in, 2 out]
      }
      frame "EIS: Start Profile" {
        n116 = local write "EIS Tab Control"(T1."RUNNING" ("EIS Tab Control")) -> ()
        n117 = Bundle By Name(cluster=w320, "EIS Profile State"=enum16{"Idle", "Start", "Run", "Stop"}."Start") -> (w319:T5)
      }
      frame "EIS: Stop Profile" {
        n118 = Bundle By Name(cluster=w325, "EIS Profile State"=enum16{"Idle", "Start", "Run", "Stop"}."Stop") -> (w324:T5)
      }
      frame "EIS: Profile Complete" {
        n119 = Unbundle By Name(w332) -> ("Profile Complete Event"=w337:refnum<user-event>, "EIS TDMS Path"=w330:path)
        n120 = Path To String(path=w330) -> (string=w329:string)
        n121 = Format Into String(format string="EIS Profile data saved to %s" ("event data"), w329) -> (resulting string=w335:string)  [unwired: 2 in, 1 out]
        n122 = Generate User Event(user event=w337, event data cluster=w335, error in=w334) -> (error out=w333:errorcluster)  [unwired: 1 in, 1 out]
        n123 = Bundle By Name(cluster=w332, "EIS Profile State"=enum16{"Idle", "Start", "Run", "Stop"}."Idle") -> (w331:T5)
      }
      frame "EIS: Generate Plots" {
        n124 = Unbundle By Name(w348) -> ("EIS TDMS Path"=w347:path, "EIS Parameters"=w339:T4)
        n125 = call "Generate EIS Plots.vi"("error in (no error)"=w346, "EIS Parameters"=w339, "TDMS Data File"=w347) -> ("error out"=w344:errorcluster, "EIS Bode Magnitude"=→"EIS Magnitude":cluster{dbl[], dbl[]}, "EIS Bode Phase"=→"EIS Phase":cluster{dbl[], dbl[]}, "EIS Nyquist"=→"EIS Nyquist":cluster{dbl[], dbl[]})  [unwired: 5 in]
        n126 = local write "EIS Tab Control"(T1."NYQUIST" ("EIS Tab Control")) -> ()
        n127 = property on="Save EIS Report" class="Bool"("DisabledEnum"=T6."Enabled" ("Disabled")) -> ()  [unwired: 2 in, 2 out]
      }
      frame "EIS: Save Report" {
        n128 = disable-structure shown="TARGET_TYPE==Windows, Default" {
          disable-tunnel: w352 -> [w363 w418]
          disable-tunnel: w351 -> [w357 _]
          disable-tunnel: [w355 w418] -> w350
          frame condition #0 (active) {
            n129 = call "File Dialog"("error in"=w363, "pattern (all files)"="*.html", "pattern label"="HTML Report") -> ("selected path"=w356:path, "cancelled"=w360:bool, "error out"=w358:errorcluster)  [unwired: 9 in, 1 out]
            n130 = Or(x=w360, y=w358) -> (x .or. y?=w359:bool)
            n131 = case shown="False" w359 {
              tunnel: w358 -> [w415 w417]
              tunnel: w357 -> [w410 _]
              tunnel: w356 -> [w403 _]
              tunnel: [w397 w417] -> w355
              frame False {
                w401 = enum16{".jpg", ".png"}.".png" ("image file type (.jpg)")
                n132 = property on="Running Status Log" class="LstBox (strict)"() -> ("Item Names"=w400:string[])  [unwired: 2 in, 2 out]
                n133 = call <vilib>:"Create Report.vi"("report type"=Report_Type."HTML", "error in (no error)"=w415) -> ("report out"=w413:refnum<class "NI_report.lvclass">, "error out"=w414:errorcluster)  [unwired: 12 in]
                n134 = call-dynamic "Set Report Header Text.vi"("report in"=w413, "left header text"="HPS17K Panel", "center header text"="EIS Report", "right header text"=w410, "error in (no error)"=w414) -> ("report out"=w386:refnum<class "NI_report.lvclass">, "error out"=w387:errorcluster)  [unwired: 9 in]
                n135 = call-dynamic "Append Horizontal Line to Report.vi"("report in"=w386, "error in (no error)"=w387) -> ("report out"=w384:refnum<class "NI_report.lvclass">, "error out"=w385:errorcluster)  [unwired: 12 in]
                n136 = control-ref of="EIS Profile"() -> (w396:refnum<vi>)
                n137 = call-dynamic "Append List to Report.vi"("report in"=w384, "list elements"=w400, "error in (no error)"=w385) -> ("report out"=w382:refnum<class "NI_report.lvclass">, "error out"=w383:errorcluster)  [unwired: 9 in, 2 out]
                n138 = control-ref of="EIS Magnitude"() -> (w406:refnum<vi>)
                n139 = control-ref of="EIS Phase"() -> (w407:refnum<vi>)
                n140 = control-ref of="EIS Nyquist"() -> (w408:refnum<vi>)
                n141 = control-ref of="EIS Parameters"() -> (w388:refnum<vi>)
                n142 = call-dynamic "Append Horizontal Line to Report.vi"("report in"=w382, "error in (no error)"=w383) -> ("report out"=w380:refnum<class "NI_report.lvclass">, "error out"=w381:errorcluster)  [unwired: 12 in]
                n143 = call-dynamic "Append Control Image to Report.vi"("report in"=w380, "ctrl reference"=w388, "description"="EIS Parameters", "error in (no error)"=w381) -> ("report out"=w378:refnum<class "NI_report.lvclass">, "error out"=w379:errorcluster)  [unwired: 8 in, 2 out]
                n144 = call-dynamic "Append Horizontal Line to Report.vi"("report in"=w378, "error in (no error)"=w379) -> ("report out"=w376:refnum<class "NI_report.lvclass">, "error out"=w377:errorcluster)  [unwired: 12 in]
                n145 = call-dynamic "Append Control Image to Report.vi"("report in"=w376, "image file type (.jpg)"=w401, "ctrl reference"=w396, "description"="EIS Profile", "error in (no error)"=w377) -> ("report out"=w374:refnum<class "NI_report.lvclass">, "error out"=w375:errorcluster)  [unwired: 7 in, 2 out]
                n146 = call-dynamic "Append Horizontal Line to Report.vi"("report in"=w374, "error in (no error)"=w375) -> ("report out"=w372:refnum<class "NI_report.lvclass">, "error out"=w373:errorcluster)  [unwired: 12 in]
                n147 = call-dynamic "Append Control Image to Report.vi"("report in"=w372, "image file type (.jpg)"=w401, "ctrl reference"=w408, "description"="EIS Nyquist", "error in (no error)"=w373) -> ("report out"=w370:refnum<class "NI_report.lvclass">, "error out"=w371:errorcluster)  [unwired: 7 in, 2 out]
                n148 = call-dynamic "Append Horizontal Line to Report.vi"("report in"=w370, "error in (no error)"=w371) -> ("report out"=w368:refnum<class "NI_report.lvclass">, "error out"=w369:errorcluster)  [unwired: 12 in]
                n149 = call-dynamic "Append Control Image to Report.vi"("report in"=w368, "image file type (.jpg)"=w401, "ctrl reference"=w407, "description"="EIS Phase", "error in (no error)"=w369) -> ("report out"=w367:refnum<class "NI_report.lvclass">, "error out"=w364:errorcluster)  [unwired: 7 in, 2 out]
                n150 = call-dynamic "Append Horizontal Line to Report.vi"("report in"=w367, "error in (no error)"=w364) -> ("report out"=w366:refnum<class "NI_report.lvclass">, "error out"=w365:errorcluster)  [unwired: 12 in]
                n151 = call-dynamic "Append Control Image to Report.vi"("report in"=w366, "image file type (.jpg)"=w401, "ctrl reference"=w406, "description"="EIS Magnitude", "error in (no error)"=w365) -> ("report out"=w394:refnum<class "NI_report.lvclass">, "error out"=w395:errorcluster)  [unwired: 7 in, 2 out]
                n152 = call-dynamic "Append User Formatted HTML to Report.vi"("report in"=w394, "HTML text"="<style>body {background-color:#111111;color:#ECECED}</style>", "error in (no error)"=w395) -> ("report out"=w392:refnum<class "NI_report.lvclass">, "error out"=w393:errorcluster)  [unwired: 11 in]
                n153 = call-dynamic "Save Report to File.vi"("report in"=w392, "report file path"=w403, "prompt to replace? (F)"=TRUE, "error in (no error)"=w393) -> ("report out"=w399:refnum<class "NI_report.lvclass">, "error out"=w398:errorcluster)  [unwired: 10 in]
                n154 = call-poly <vilib>:"Open HTML Report in Browser.vi"("report in"=w399, "error in (no error)"=w398) -> ("error out"=w397:errorcluster)  [unwired: 11 in, 2 out]
              }
              frame True {
              }
            }
          }
          frame condition #1 {
          }
        }
      }
      frame "---------- UI ----------" {
      }
      frame "UI: Front Panel State" {
        n155 = case shown="\"Close\"" w423 {
          frame "Open", Default {
            n156 = property class="VI"() -> ("FP.State"=w426:T8)  [unwired: 2 in, 2 out]
            n157 = case shown="Default" w426 {
              frame Default {
                n158 = invoke class="VI" method="FP.Open"("Activate"=TRUE, "State"=T8."Standard") -> ()  [unwired: 3 in, 5 out]
              }
              frame "Standard" {
              }
            }
          }
          frame "Close" {
            n159 = property class="VI"() -> ("FP.State"=w429:T8)  [unwired: 2 in, 2 out]
            n160 = case shown="Default" w429 {
              frame "Closed" {
              }
              frame Default {
                n161 = invoke class="VI" method="FP.Close"() -> ()  [unwired: 3 in, 3 out]
              }
            }
          }
        }
      }
      frame "UI: Initialize" {
        w431 = cluster{dbl[], dbl[]} {[], []} ("EIS Nyquist")
        n162 = property class="VI"() -> ("Name"=w446:string)  [unwired: 2 in, 2 out]
        n163 = Match Pattern(string=w446, regular expression="\\2Evi$") -> (before substring=w444:string)  [unwired: 1 in, 3 out]
        n164 = local write "EIS Tab Control"(T1."PROFILE" ("EIS Tab Control")) -> ()
        n165 = property on="Running Status Log" class="LstBox (strict)"("Item Names"=string[] []) -> ()  [unwired: 2 in, 2 out]
        n166 = Reverse String(1:w444) -> (0:w443:string)
        n167 = Match Pattern(string=w443, regular expression=":") -> (before substring=w441:string, after substring=w440:string)  [unwired: 1 in, 2 out]
        n168 = local write "EIS Profile"(waveform(dbl)[] [] ("EIS Profile")) -> ()
        n169 = local write "EIS Magnitude"(w431) -> ()
        n170 = local write "EIS Phase"(w431) -> ()
        n171 = local write "EIS Nyquist"(w431) -> ()
        n172 = Match Pattern(string=w440, regular expression="\\2E") -> (after substring=w438:string)  [unwired: 1 in, 3 out]
        n173 = Reverse String(1:w438) -> (0:w437:string)
        n174 = Reverse String(1:w441) -> (0:w436:string)
        n175 = Format Into String(format string="%s %s", w437, w436) -> (resulting string=w435:string)  [unwired: 2 in, 1 out]
        n176 = property class="VI"("Front Panel.Title"=w435) -> ()  [unwired: 2 in, 2 out]
        n177 = property on="Save EIS Report" class="Bool"("DisabledEnum"=T6."Disabled and Grayed Out" ("Disabled")) -> ()  [unwired: 2 in, 2 out]
      }
      frame "UI: Cleanup" {
        n178 = property class="VI"() -> (error out=w451:errorcluster, "FP.State"=w453:T8)  [unwired: 2 in, 1 out]
        n179 = case shown="\"Standard\", Default" w453 {
          frame "Closed" {
          }
          frame "Standard", Default {
            n180 = invoke class="VI" method="FP.Close"() -> ()  [unwired: 3 in, 3 out]
          }
        }
      }
      frame "---------- CMD ----------" {
      }
      frame "CMD: Exit" {
      }
      frame "CMD: Front Panel State" {
        n181 = Format Into String(format string="UI: Front Panel State>>%s" ("string"), w462) -> (resulting string=w461:string)  [unwired: 2 in, 1 out]
        n182 = call <vilib>:"Add State(s) to Queue__jki_lib_state_machine.vi"("State(s) in (\"\")"=w465, "State(s) at Back (\"\")"=w461) -> ("States Out"=w464:string)  [unwired: 13 in]
      }
      frame "CMD: Start Profile" {
        n183 = Unbundle By Name(w473) -> ("Profile Complete Event"=w476:refnum<user-event>, "Core.Data"=w477:variant)
        n184 = call <vilib>:"Add State(s) to Queue__jki_lib_state_machine.vi"("State(s) in Front (\"\")"="EIS: Start Profile", "State(s) in (\"\")"=w470) -> ("States Out"=w469:string)  [unwired: 13 in]
        n185 = Variant To Data(error in=w475, type=w476, Variant=w477) -> (data=w471:refnum<user-event>, error out=w474:errorcluster)
        n186 = Bundle By Name(cluster=w473, "Profile Complete Event"=w471) -> (w472:T5)
      }
      frame "CMD: Generate Plots" {
        n187 = call <vilib>:"Add State(s) to Queue__jki_lib_state_machine.vi"("State(s) in Front (\"\")"="EIS: Generate Plots", "State(s) in (\"\")"=w480) -> ("States Out"=w479:string)  [unwired: 13 in]
      }
      frame "CMD: Stop Profile" {
        n188 = call <vilib>:"Add State(s) to Queue__jki_lib_state_machine.vi"("State(s) in Front (\"\")"="EIS: Stop Profile", "State(s) in (\"\")"=w484) -> ("States Out"=w483:string)  [unwired: 13 in]
      }
    }
  }
  "error out" <- w4
  "reference out" <- "reference in"
